vi "6.vi"() -> ()   [LabVIEW 2017]
uses:
  <vilib>/measure/NI_MABase.lvlib
panel:
  out "大小":i32
  out "最大值":dbl
  out "dt":dbl
  in  "sampling info":cluster{"Fs":dbl, "#s":dbl}={"Fs"=1000.0, "#s"=1000.0} caption="采样信息" {"Fs" format="%.2p"}
  in  "phase":dbl caption="相位" format="%.2p"
  in  "amplitude":dbl=1.0 caption="幅值" format="%0.2p"
  in  "frequency":dbl=10.0 caption="频率" format="%0.2p"
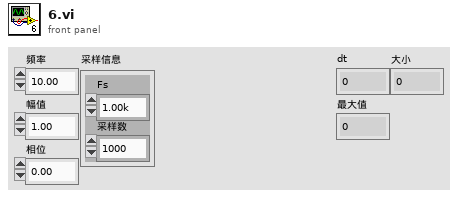
[diagram p1: front panel]
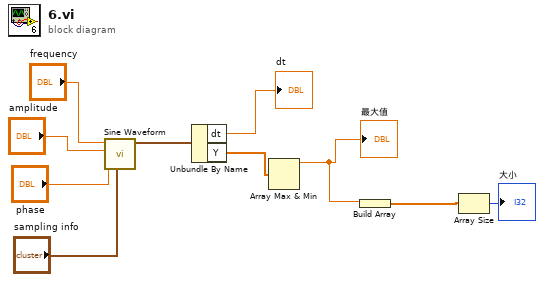
[diagram p0: block diagram]
diagram:
  n1 = call <vilib>:"Sine Waveform.vi"("sampling info"="sampling info", "phase"="phase", "amplitude"="amplitude", "frequency"="frequency") -> ("signal out"=w10:waveform(dbl))  [unwired: 6 in, 1 out]
  n2 = Unbundle By Name(w10) -> ("dt"=→"dt":dbl, "Y"=w4:dbl[])
  n3 = Array Max & Min(array=w4) -> (max value=w3:dbl)  [unwired: 3 out]
  "最大值" <- w3
  n4 = Build Array(w3) -> (w2:dbl[])
  n5 = Array Size(array=w2) -> (size(s)=→"大小":i32)
